vi "blastPulse.vi"() -> ()   [LabVIEW 2015]
doc: "The UDP protocol differs from TCP in that there is no error-checking with the packets of information that are sent, and thus no guarantee whatsoever that an intended recipient will actually receive a given piece of data.\n\nUDP does offer the ability to \"broadcast\" data across a network--simply specify an IP Address of all ones (255.255.255.255) to attempt to broadcast information network-wide. Keep in mind that routers and other network hardware will generally refuse to forward the broadcast beyond certain points, so the extent of the broadcast will in practice be limited."
panel:
  in  "Solenoid Close time (Default 0.009 Seconds)":dbl
  in  "Solenoid Idle Time (Default 0.008 Seconds)":dbl
  in  "Solenoid Open Time (Default 0.004 Seconds)":dbl
  in  "Number of Blasts":dbl
  in  "Blast Interval (s)":dbl
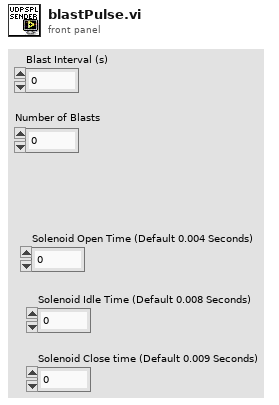
[diagram p1: front panel]
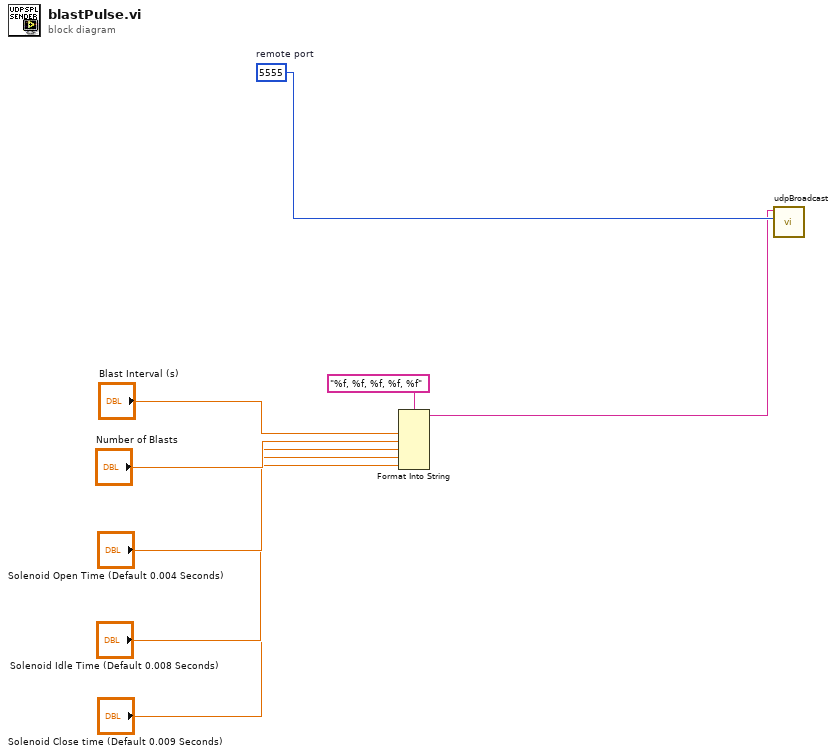
[diagram p0: block diagram]
diagram:
  w8 = u16 5555  # remote port
  n1 = Format Into String(format string="%f, %f, %f, %f, %f", "Blast Interval (s)", "Number of Blasts", "Solenoid Open Time (Default 0.004 Seconds)", "Solenoid Idle Time (Default 0.008 Seconds)", "Solenoid Close time (Default 0.009 Seconds)") -> (resulting string=w1:string)  [unwired: 2 in, 1 out]
  n2 = call "udpBroadcast.vi"("remote port"=w8, "data in"=w1) -> ()  [unwired: 10 in]
